vi "Set Reference.vi"(8 "Error In":errorcluster, 10 "Reference":refnum<class "ILogger.lvclass">, 11 "Logger In":refnum<class "LoggerAPI.lvclass">) -> (0 "Error Out":errorcluster, 3 "Logger Out":refnum<class "LoggerAPI.lvclass">)   [LabVIEW 2020, in "LoggerAPI.lvclass"]
uses:
  LoggerAPI.lvclass
  ILogger/ILogger.lvclass
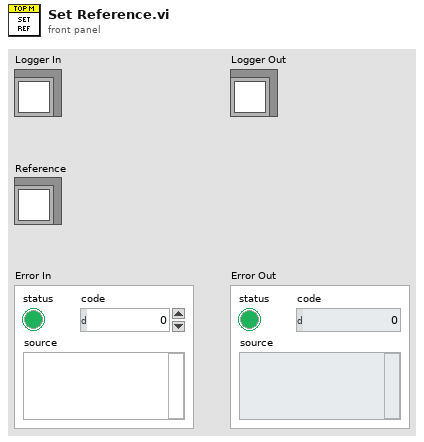
[diagram p1: front panel]
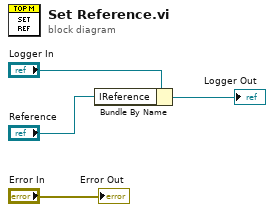
[diagram p0: block diagram]
diagram:
  n1 = Bundle By Name(cluster="Logger In", "IReference"="Reference") -> (→"Logger Out":refnum<class "LoggerAPI.lvclass">)
  "Error Out" <- "Error In"
